vi "uStringManipulation_DO.vi"(8 "error in (no error)":errorcluster, 10 "Filename in":string, 11 "in":refnum<class "SaneWinFilename.lvclass">) -> (0 "error out":errorcluster, 2 "Filename Out":string, 3 "out":refnum<class "SaneWinFilename.lvclass">)   [LabVIEW 2023, in "uLib.lvlib" / "SaneWinFilename.lvclass"]
doc: "This method cleans up the filename string from any illegal characters that are not accepted by the OS filesystem and replaces them with underscores. It executes regardless of the error-in state."
uses:
  SaneWinFilename.lvclass
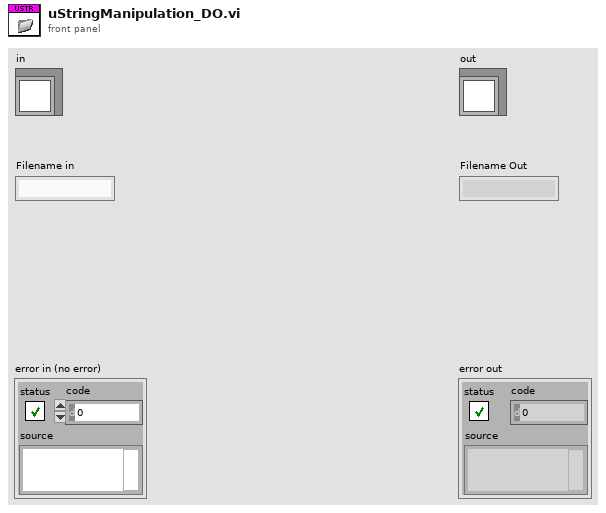
[diagram p1: front panel]
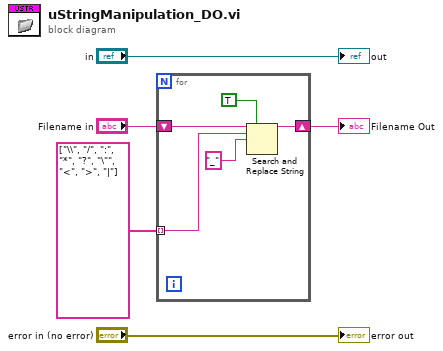
[diagram p0: block diagram]
diagram:
  n1 = for {
    shift-right: [w9] -> w1
    shift-left: "Filename in" -> [w10]
    tunnel: string[] ["\\", "/", ":", "*", "?", "\"", "<", ">", "|"] -> [w6] mode=indexing
    n2 = Search and Replace String(replace all?=TRUE ("replace all? (F)"), input string=w10, search string=w6, replace string="_" ("replace string (\"\")")) -> (result string=w9:string)  [unwired: 4 in, 3 out]
  }
  "Filename Out" <- w1
  "error out" <- "error in (no error)"
  "out" <- "in"
